vi "45-1599-1 Test.vi"() -> ()   [LabVIEW 2015]
uses:
  C:/Program Files (x86)/Hunter/Factory/QCDClean/QuickLaserFactoryCalibration.dll
  QuickLaserFactoryCalibration.dll
  <vilib>/Utility/file.llb/Write Delimited Spreadsheet (string).vi
panel:
  in  "Barcode":string
  in  "Barcode":string
  out "IR Status":u8
  out "IR FAIL":bool
  out "IR PASS":bool
  in  "START TEST":bool
  out "Test Inspection Imager FAIL":bool=TRUE
  out "Test Main Imager FAIL":bool=TRUE
  out "Laser FAIL":bool=TRUE
  out "Laser PASS":bool=TRUE
  out "Laser Status":u8
  out "Set Sync FAIL":bool=TRUE
  out "Set Sync PASS":bool=TRUE
  out "Jumpers FAIL":bool
  out "Jumpers PASS":bool
  out "Jumper Status":u8
  out "D4":bool
  out "D3":bool
  out "D2":bool
  out "D1":bool
  out "Test Inspection Imager PASS":bool
  out "Test Main Imager PASS":bool
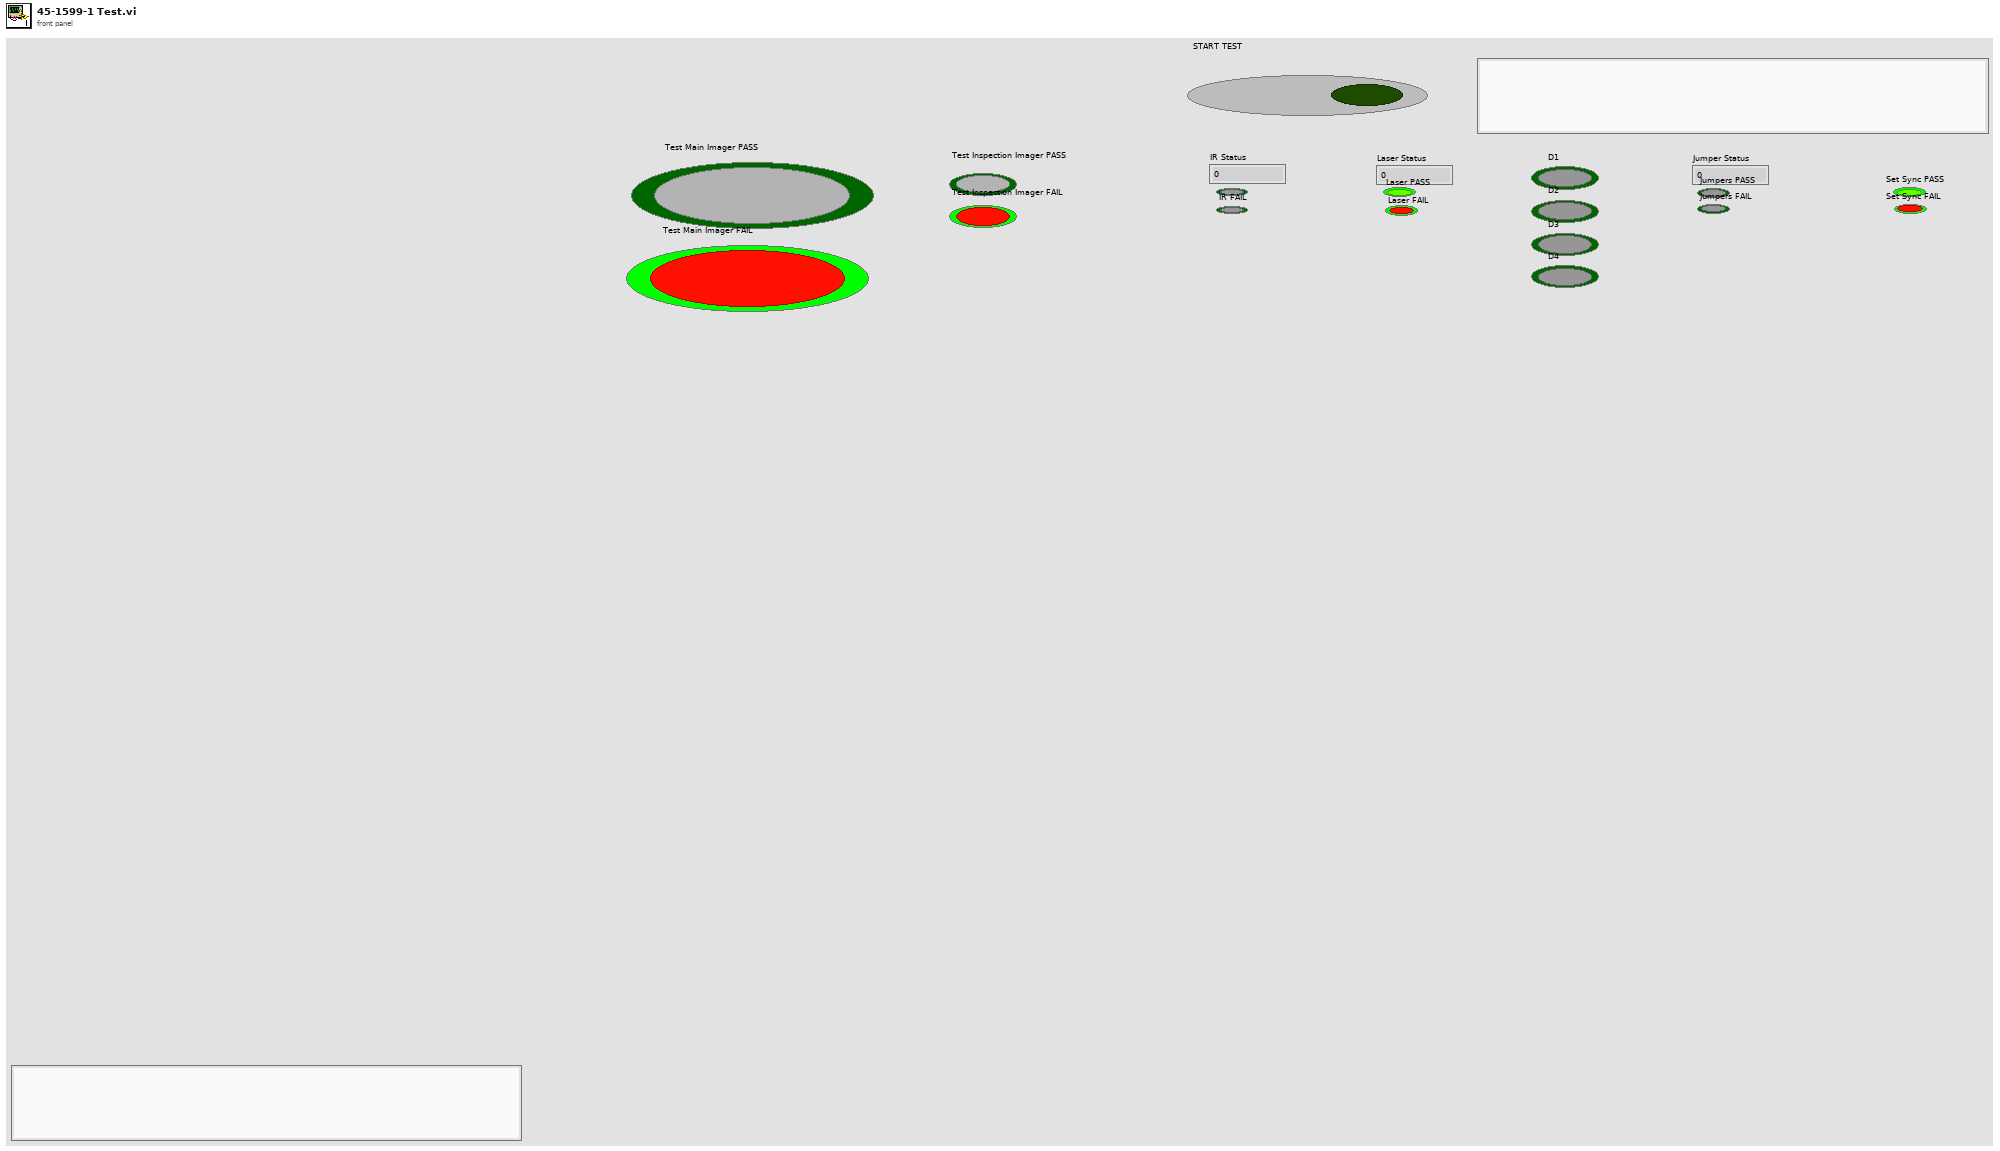
[diagram p1: front panel]
types:
  T1 = enum8{"Enabled", "Disabled", "Disabled and Grayed Out"}
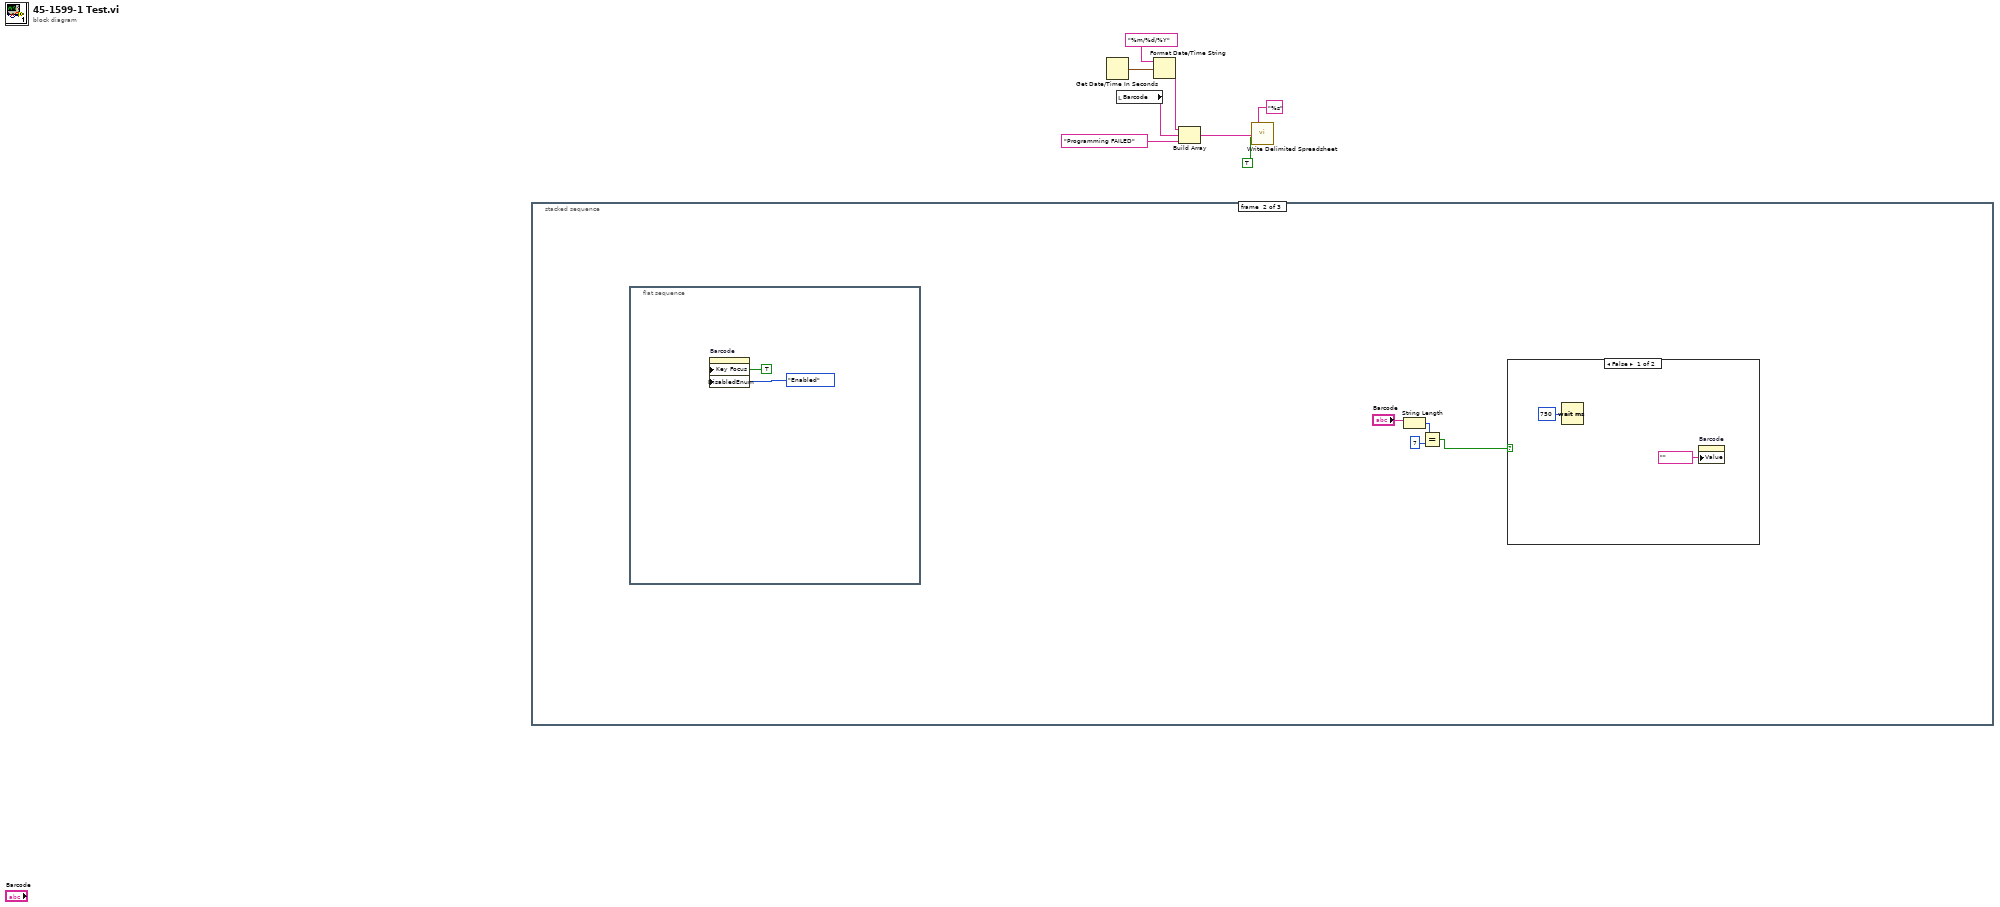
[diagram p0: block diagram]
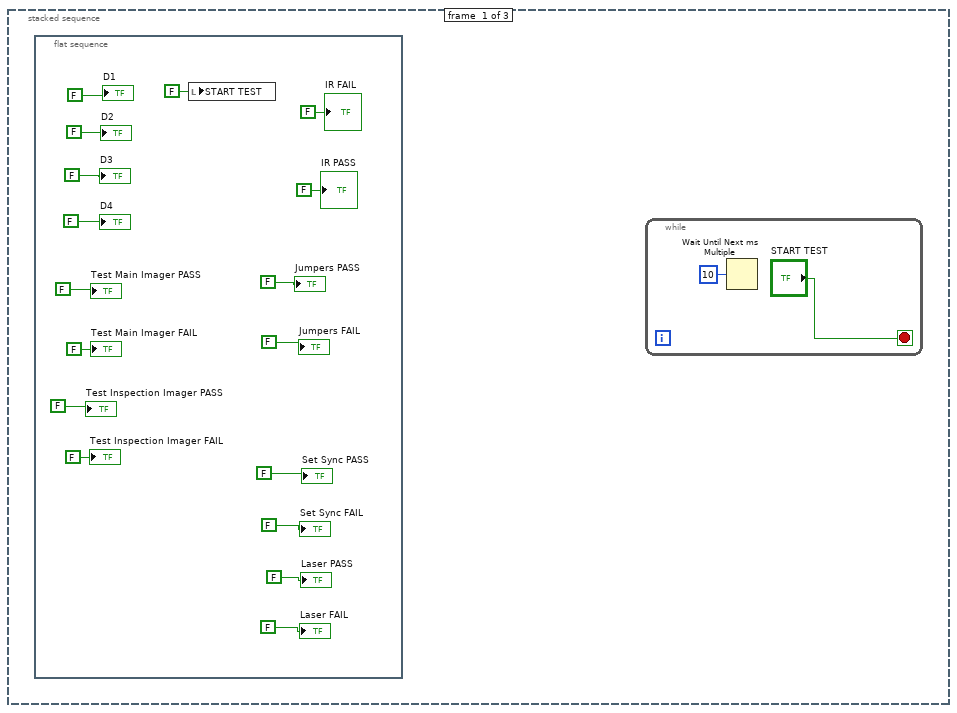
[diagram p2: hidden frame]
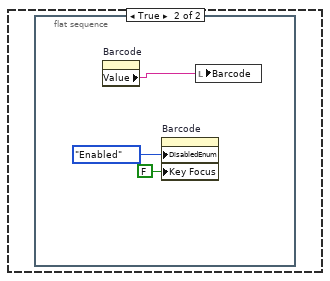
[diagram p3: hidden frame]
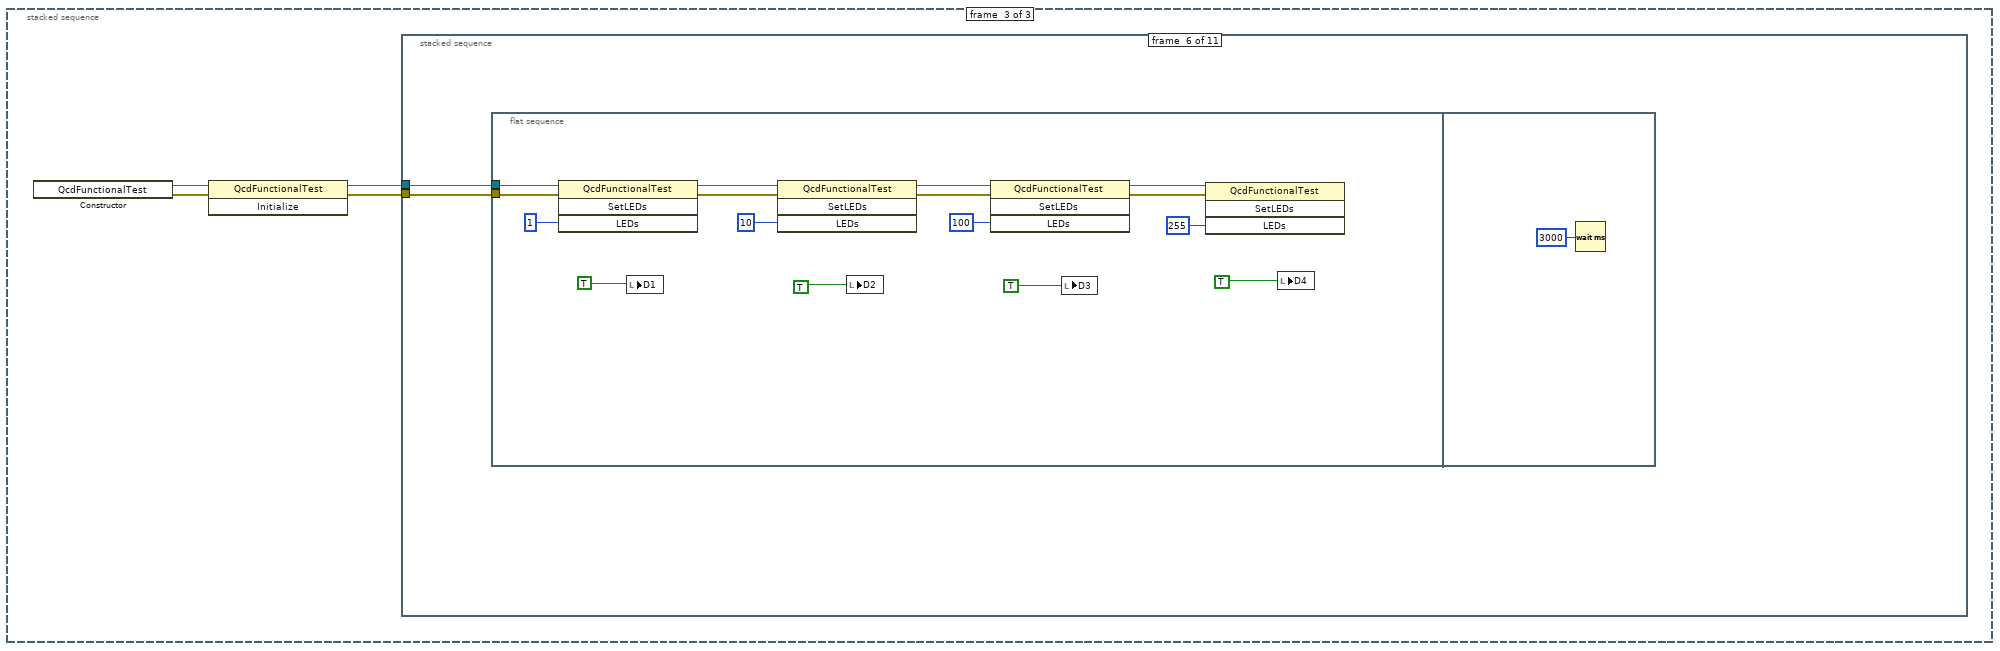
[diagram p4: hidden frame]
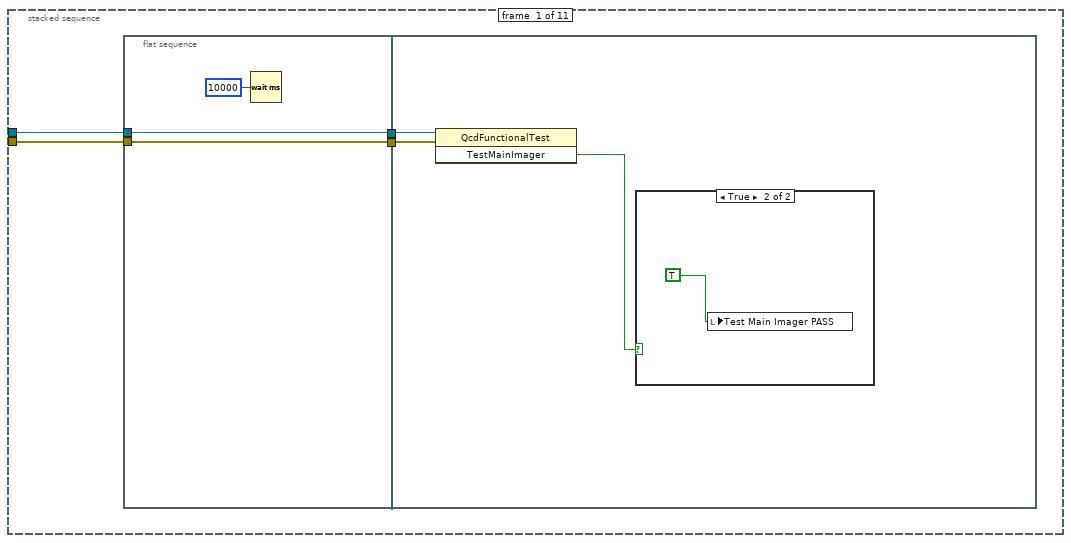
[diagram p5: hidden frame]
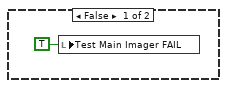
[diagram p6: hidden frame]
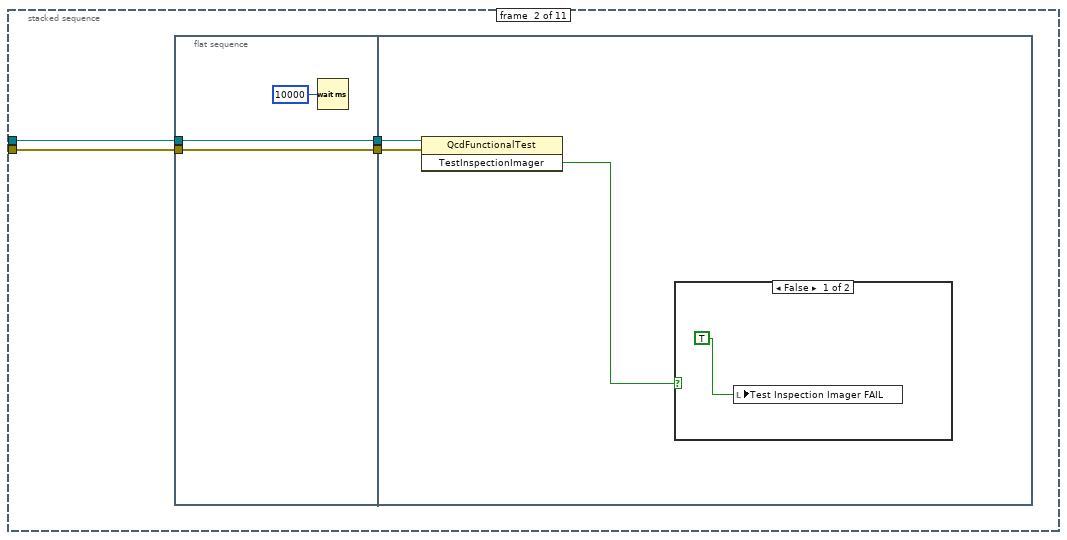
[diagram p7: hidden frame]
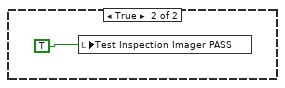
[diagram p8: hidden frame]
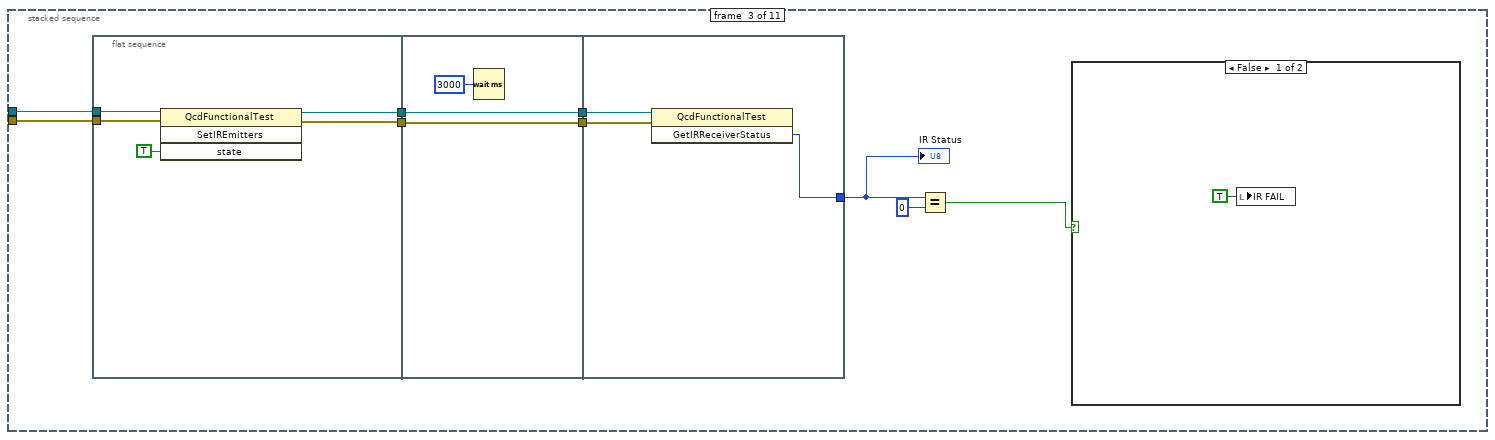
[diagram p9: hidden frame]
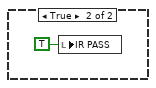
[diagram p10: hidden frame]
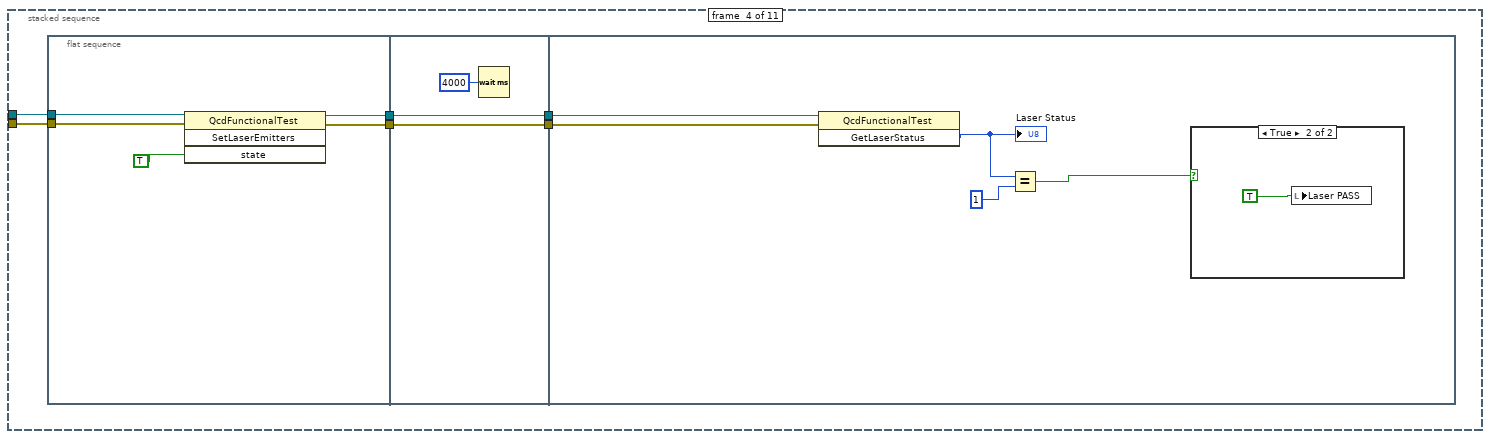
[diagram p11: hidden frame]
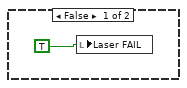
[diagram p12: hidden frame]
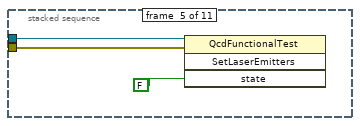
[diagram p13: hidden frame]
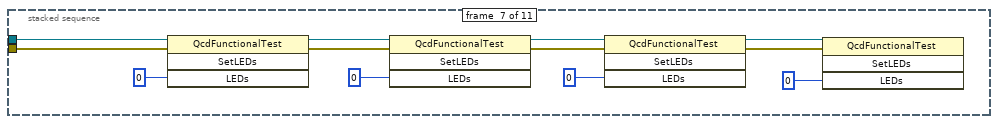
[diagram p14: hidden frame]
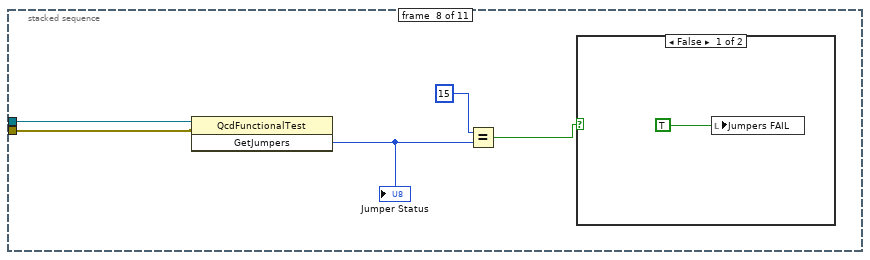
[diagram p15: hidden frame]
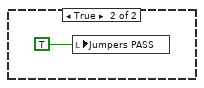
[diagram p16: hidden frame]
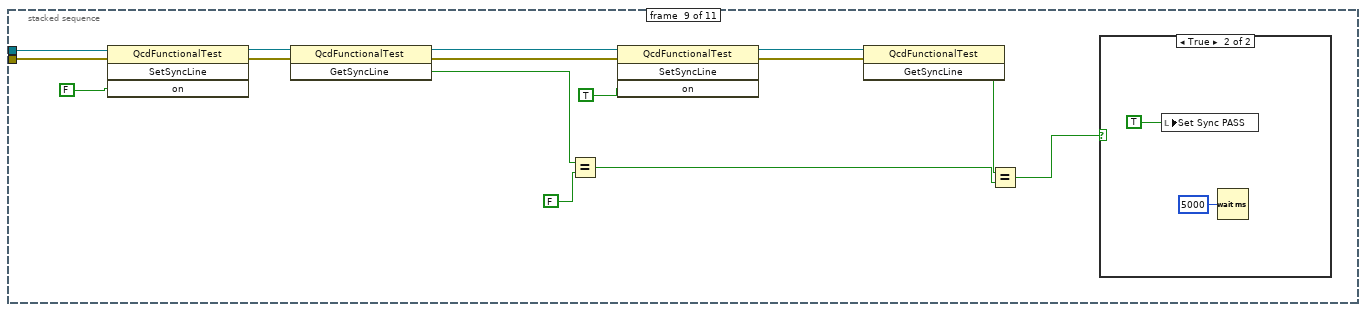
[diagram p17: hidden frame]
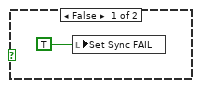
[diagram p18: hidden frame]
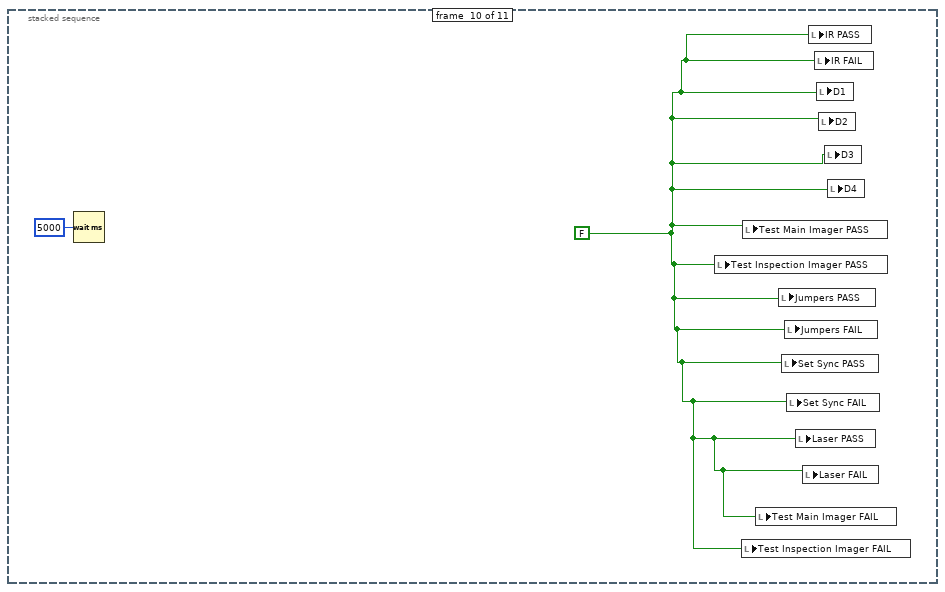
[diagram p19: hidden frame]
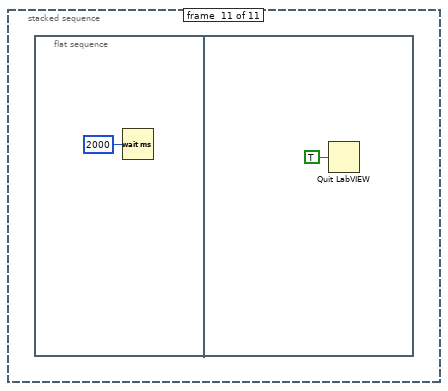
[diagram p20: hidden frame]
diagram:
  n1 = stacked-sequence {
    frame #0 {
      n2 = flat-sequence {
        frame #0 {
          n3 = local write "START TEST"(FALSE ("START TEST")) -> ()
          "D1" <- FALSE
          "D2" <- FALSE
          "D3" <- FALSE
          "D4" <- FALSE
          "IR PASS" <- FALSE ("IR PASS")
          "IR FAIL" <- FALSE ("IR FAIL")
          "Test Main Imager PASS" <- FALSE
          "Test Inspection Imager PASS" <- FALSE
          "Test Main Imager FAIL" <- FALSE ("Test Main Imager FAIL")
          "Test Inspection Imager FAIL" <- FALSE ("Test Inspection Imager FAIL")
          "Jumpers PASS" <- FALSE
          "Jumpers FAIL" <- FALSE
          "Set Sync PASS" <- FALSE
          "Set Sync FAIL" <- FALSE
          "Laser PASS" <- FALSE
          "Laser FAIL" <- FALSE
        }
      }
      n4 = while {
        stop <- "START TEST" stop-if-true
        n5 = Wait Until Next ms Multiple(millisecond multiple=u32 10) -> ()  [unwired: 1 out]
      }
    }
    frame #1 {
      n6 = flat-sequence {
        frame #0 {
          n7 = property on="Barcode" class="Str"("Key Focus"=TRUE, "DisabledEnum"=T1."Enabled" ("Disabled")) -> ()  [unwired: 2 in, 2 out]
        }
      }
      n8 = String Length(string="Barcode") -> (length=w31:i32)
      n9 = Equal?(x=w31, y=7) -> (x = y?=w29:bool)
      n10 = case shown="False" w29 {
        frame False {
          n11 = Wait (ms)(milliseconds to wait=u32 750) -> ()  [unwired: 1 out]
          n12 = property on="Barcode" class="Str"("Value"="" ("Barcode")) -> ()  [unwired: 2 in, 2 out]
        }
        frame True {
          n13 = flat-sequence {
            frame #0 {
              n14 = property on="Barcode" class="Str"() -> ("Value"=w39:string)  [unwired: 2 in, 2 out]
              n15 = property on="Barcode" class="Str"("DisabledEnum"=T1."Enabled" ("Disabled"), "Key Focus"=FALSE) -> ()  [unwired: 2 in, 2 out]
              n16 = local write "Barcode"(w39) -> ()
            }
          }
        }
      }
    }
    frame #2 {
      n17 = constructor class="QcdFunctionalTest"() -> (reference out=w42:refnum<k24>, error out=w43:errorcluster)  [unwired: 3 in, 1 out]
      n18 = invoke class="QcdFunctionalTest" method="Initialize"(reference=w42, error in=w43) -> (reference out=w41:refnum<k24>, error out=w40:errorcluster)  [unwired: 1 in, 1 out]
      n19 = stacked-sequence {
        tunnel: w41 -> [w45 w58 w76 w95 w113 w115 w144 w149 w166 _ _]
        tunnel: w40 -> [w44 w56 w75 w94 w112 w114 w143 w148 w165 _ _]
        frame #0 {
          n20 = flat-sequence {
            tunnel: [w50] -> w47
            tunnel: [w49] -> w46
            tunnel: w45 -> [w50]
            tunnel: w44 -> [w49]
            tunnel: w47 -> [w53]
            tunnel: w46 -> [w52]
            frame #0 {
              n21 = Wait (ms)(milliseconds to wait=u32 10000) -> ()  [unwired: 1 out]
            }
            frame #1 {
              n22 = invoke class="QcdFunctionalTest" method="TestMainImager"(reference=w53, error in=w52) -> ("TestMainImager"=w51:bool)  [unwired: 1 in, 2 out]
              n23 = case shown="True" w51 {
                frame False {
                  n24 = local write "Test Main Imager FAIL"(TRUE ("Test Main Imager FAIL")) -> ()
                }
                frame True {
                  n25 = local write "Test Main Imager PASS"(TRUE) -> ()
                }
              }
            }
          }
        }
        frame #1 {
          n26 = flat-sequence {
            tunnel: [w62] -> w59
            tunnel: w58 -> [w62]
            tunnel: [w61] -> w57
            tunnel: w56 -> [w61]
            tunnel: w59 -> [w64]
            tunnel: w57 -> [w63]
            frame #0 {
              n27 = Wait (ms)(milliseconds to wait=u32 10000) -> ()  [unwired: 1 out]
            }
            frame #1 {
              n28 = invoke class="QcdFunctionalTest" method="TestInspectionImager"(reference=w64, error in=w63) -> ("TestInspectionImager"=w65:bool)  [unwired: 1 in, 2 out]
              n29 = case shown="False" w65 {
                frame False {
                  n30 = local write "Test Inspection Imager FAIL"(TRUE) -> ()
                }
                frame True {
                  n31 = local write "Test Inspection Imager PASS"(TRUE) -> ()
                }
              }
            }
          }
        }
        frame #2 {
          n32 = flat-sequence {
            tunnel: w76 -> [w83]
            tunnel: w75 -> [w82]
            tunnel: [w80] -> w73
            tunnel: [w79] -> w71
            tunnel: [w85] -> w74
            tunnel: w73 -> [w85]
            tunnel: [w84] -> w72
            tunnel: w71 -> [w84]
            tunnel: w74 -> [w89]
            tunnel: w72 -> [w88]
            tunnel: [w87] -> w68
            frame #0 {
              n33 = invoke class="QcdFunctionalTest" method="SetIREmitters"(reference=w83, error in=w82, "state"=TRUE) -> (reference out=w80:refnum<k24>, error out=w79:errorcluster)  [unwired: 1 in, 2 out]
            }
            frame #1 {
              n34 = Wait (ms)(milliseconds to wait=u32 3000) -> ()  [unwired: 1 out]
            }
            frame #2 {
              n35 = invoke class="QcdFunctionalTest" method="GetIRReceiverStatus"(reference=w89, error in=w88) -> ("GetIRReceiverStatus"=w87:u8)  [unwired: 1 in, 2 out]
            }
          }
          n36 = Equal?(x=w68, y=u8 0) -> (x = y?=w69:bool)
          n37 = case shown="False" w69 {
            frame False {
              n38 = local write "IR FAIL"(TRUE ("IR FAIL")) -> ()
            }
            frame True {
              n39 = local write "IR PASS"(TRUE ("IR PASS")) -> ()
            }
          }
          "IR Status" <- w68
        }
        frame #3 {
          n40 = flat-sequence {
            tunnel: w94 -> [w98]
            tunnel: w95 -> [w99]
            tunnel: [w97] -> w93
            tunnel: [w96] -> w91
            tunnel: w93 -> [w103]
            tunnel: [w103] -> w92
            tunnel: w91 -> [w102]
            tunnel: [w102] -> w90
            tunnel: w92 -> [w105]
            tunnel: w90 -> [w104]
            frame #0 {
              n41 = invoke class="QcdFunctionalTest" method="SetLaserEmitters"(reference=w99, error in=w98, "state"=TRUE) -> (reference out=w97:refnum<k24>, error out=w96:errorcluster)  [unwired: 1 in, 2 out]
            }
            frame #1 {
              n42 = Wait (ms)(milliseconds to wait=u32 4000) -> ()  [unwired: 1 out]
            }
            frame #2 {
              n43 = invoke class="QcdFunctionalTest" method="GetLaserStatus"(reference=w105, error in=w104) -> ("GetLaserStatus"=w108:u8)  [unwired: 1 in, 2 out]
              "Laser Status" <- w108
              n44 = Equal?(x=w108, y=u8 1) -> (x = y?=w106:bool)
              n45 = case shown="True" w106 {
                frame False {
                  n46 = local write "Laser FAIL"(TRUE) -> ()
                }
                frame True {
                  n47 = local write "Laser PASS"(TRUE) -> ()
                }
              }
            }
          }
        }
        frame #4 {
          n48 = invoke class="QcdFunctionalTest" method="SetLaserEmitters"(reference=w113, error in=w112, "state"=FALSE) -> ()  [unwired: 1 in, 4 out]
        }
        frame #5 {
          n49 = flat-sequence {
            tunnel: w115 -> [w131]
            tunnel: w114 -> [w130]
            frame #0 {
              n50 = invoke class="QcdFunctionalTest" method="SetLEDs"(reference=w131, error in=w130, "LEDs"=u8 1) -> (reference out=w128:refnum<k24>, error out=w127:errorcluster)  [unwired: 1 in, 2 out]
              n51 = local write "D1"(TRUE) -> ()
              n52 = invoke class="QcdFunctionalTest" method="SetLEDs"(reference=w128, error in=w127, "LEDs"=u8 10) -> (reference out=w125:refnum<k24>, error out=w124:errorcluster)  [unwired: 1 in, 2 out]
              n53 = local write "D2"(TRUE) -> ()
              n54 = invoke class="QcdFunctionalTest" method="SetLEDs"(reference=w125, error in=w124, "LEDs"=u8 100) -> (reference out=w123:refnum<k24>, error out=w122:errorcluster)  [unwired: 1 in, 2 out]
              n55 = local write "D3"(TRUE) -> ()
              n56 = invoke class="QcdFunctionalTest" method="SetLEDs"(reference=w123, error in=w122, "LEDs"=u8 255) -> ()  [unwired: 1 in, 4 out]
              n57 = local write "D4"(TRUE) -> ()
            }
            frame #1 {
              n58 = Wait (ms)(milliseconds to wait=u32 3000) -> ()  [unwired: 1 out]
            }
          }
        }
        frame #6 {
          n59 = invoke class="QcdFunctionalTest" method="SetLEDs"(reference=w144, error in=w143, "LEDs"=u8 0) -> (reference out=w141:refnum<k24>, error out=w140:errorcluster)  [unwired: 1 in, 2 out]
          n60 = invoke class="QcdFunctionalTest" method="SetLEDs"(reference=w141, error in=w140, "LEDs"=u8 0) -> (reference out=w138:refnum<k24>, error out=w137:errorcluster)  [unwired: 1 in, 2 out]
          n61 = invoke class="QcdFunctionalTest" method="SetLEDs"(reference=w138, error in=w137, "LEDs"=u8 0) -> (reference out=w136:refnum<k24>, error out=w135:errorcluster)  [unwired: 1 in, 2 out]
          n62 = invoke class="QcdFunctionalTest" method="SetLEDs"(reference=w136, error in=w135, "LEDs"=u8 0) -> ()  [unwired: 1 in, 4 out]
        }
        frame #7 {
          n63 = invoke class="QcdFunctionalTest" method="GetJumpers"(reference=w149, error in=w148) -> ("GetJumpers"=w147:u8)  [unwired: 1 in, 2 out]
          "Jumper Status" <- w147
          n64 = Equal?(x=u8 15, y=w147) -> (x = y?=w145:bool)
          n65 = case shown="False" w145 {
            frame False {
              n66 = local write "Jumpers FAIL"(TRUE) -> ()
            }
            frame True {
              n67 = local write "Jumpers PASS"(TRUE) -> ()
            }
          }
        }
        frame #8 {
          n68 = invoke class="QcdFunctionalTest" method="SetSyncLine"(reference=w166, error in=w165, "on"=FALSE) -> (reference out=w163:refnum<k24>, error out=w162:errorcluster)  [unwired: 1 in, 2 out]
          n69 = invoke class="QcdFunctionalTest" method="GetSyncLine"(reference=w163, error in=w162) -> (reference out=w161:refnum<k24>, error out=w160:errorcluster, "GetSyncLine"=w156:bool)  [unwired: 1 in]
          n70 = Equal?(x=w156, y=FALSE) -> (x = y?=w154:bool)
          n71 = invoke class="QcdFunctionalTest" method="SetSyncLine"(reference=w161, error in=w160, "on"=TRUE) -> (reference out=w159:refnum<k24>, error out=w158:errorcluster)  [unwired: 1 in, 2 out]
          n72 = invoke class="QcdFunctionalTest" method="GetSyncLine"(reference=w159, error in=w158) -> ("GetSyncLine"=w153:bool)  [unwired: 1 in, 2 out]
          n73 = Equal?(x=w153, y=w154) -> (x = y?=w152:bool)
          n74 = case shown="True" w152 {
            frame False {
              n75 = local write "Set Sync FAIL"(TRUE) -> ()
            }
            frame True {
              n76 = local write "Set Sync PASS"(TRUE) -> ()
              n77 = Wait (ms)(milliseconds to wait=u32 5000) -> ()  [unwired: 1 out]
            }
          }
        }
        frame #9 {
          w170 = FALSE
          n78 = Wait (ms)(milliseconds to wait=u32 5000) -> ()  [unwired: 1 out]
          n79 = local write "Test Inspection Imager PASS"(w170) -> ()
          n80 = local write "Test Inspection Imager FAIL"(w170) -> ()
          n81 = local write "Test Main Imager PASS"(w170) -> ()
          n82 = local write "Test Main Imager FAIL"(w170) -> ()
          n83 = local write "Jumpers PASS"(w170) -> ()
          n84 = local write "Set Sync PASS"(w170) -> ()
          n85 = local write "Jumpers FAIL"(w170) -> ()
          n86 = local write "Set Sync FAIL"(w170) -> ()
          n87 = local write "Laser PASS"(w170) -> ()
          n88 = local write "Laser FAIL"(w170) -> ()
          n89 = local write "IR PASS"(w170) -> ()
          n90 = local write "IR FAIL"(w170) -> ()
          n91 = local write "D1"(w170) -> ()
          n92 = local write "D2"(w170) -> ()
          n93 = local write "D3"(w170) -> ()
          n94 = local write "D4"(w170) -> ()
        }
        frame #10 {
          n95 = flat-sequence {
            frame #0 {
              n96 = Wait (ms)(milliseconds to wait=u32 2000) -> ()  [unwired: 1 out]
            }
            frame #1 {
              n97 = Quit LabVIEW(quit? (T)=TRUE) -> ()
            }
          }
        }
      }
    }
  }
  n98 = Get Date/Time In Seconds() -> (seconds since 1Jan1904=w6:timestamp)
  n99 = local read "Barcode"() -> (w3:string)
  n100 = Format Date/Time String(time format string (%c)="%m/%d/%Y", seconds (now)=w6) -> (date/time string=w4:string)  [unwired: 1 in]
  n101 = Build Array(w4, w3, "Programming FAILED" ("element")) -> (w7:string[])
  n102 = call-poly <vilib>:"Write Delimited Spreadsheet.vi"("format (%s)"="%s" ("format (%.3f)"), "1D data"=w7, "append to file? (F)"=TRUE) -> ("file path (dialog if empty)"=w1:path)  [unwired: 10 in, 2 out]
